vi "Get Reference for Specified Type (Project).vi"(8 "error in (no error)":errorcluster, 10 "Type to Find":string, 11 "Array of References":refnum<vi>[](array[refnum])) -> (0 "error out":errorcluster, 2 "Item Found":bool, 3 "Project Item":refnum<vi>)   [LabVIEW 2014, in "SPI Engine Scripting.lvlib"]
uses:
  SPI Engine Scripting.lvlib
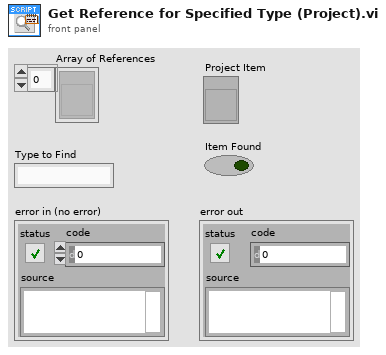
[diagram p1: front panel]
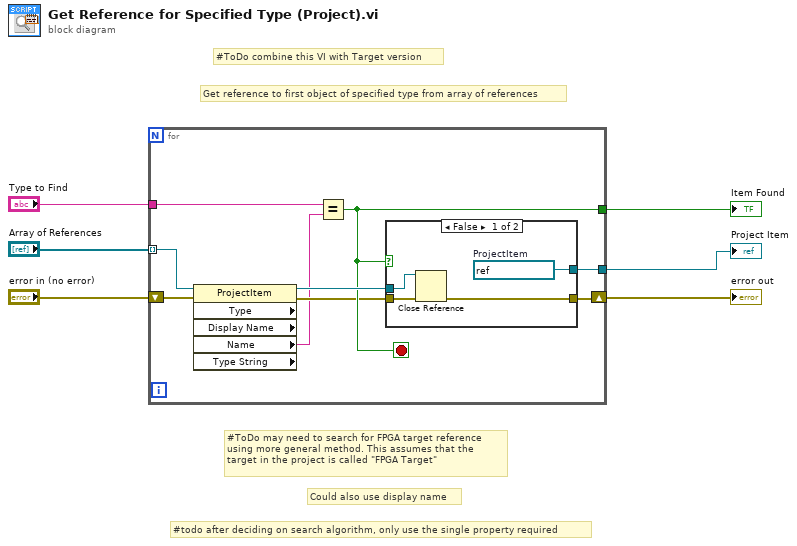
[diagram p0: block diagram]
diagram:
  # "#todo after deciding on search algorithm, only use the single property required"
  # "#ToDo combine this VI with Target version"
  # "#ToDo may need to search for FPGA target reference\nusing more general method. This assumes that the\ntarget in the project is called \"FPGA Target\""
  # "Could also use display name"
  # "Get reference to first object of specified type from array of references"
  n1 = for {
    tunnel: "Array of References" -> [w15] mode=indexing
    tunnel: "Type to Find" -> [w12]
    tunnel: [w11] -> w2
    shift-right: [w9] -> w3
    shift-left: "error in (no error)" -> [w14]
    tunnel: [w8] -> w1
    stop <- w11 stop-if-true
    n2 = property class="ProjectItem" props=["Type", "Display Name", "Name", "Type String"](reference=w15, error in=w14) -> (reference out=w13:refnum<vi>, error out=w10:errorcluster, "Name"=w7:string)  [unwired: 3 out]
    n3 = Equal?(x=w12, y=w7) -> (x = y?=w11:bool)
    n4 = case shown="False" w11 {
      tunnel: w13 -> [w17 w21]
      tunnel: [w16 w21] -> w8
      tunnel: w10 -> [w19 w20]
      tunnel: [w18 w20] -> w9
      frame False {
        w16 = refnum<vi> refnum  # ProjectItem
        n5 = Close Reference(reference=w17, error in (no error)=w19) -> (error out=w18:errorcluster)
      }
      frame True {
      }
    }
  }
  "error out" <- w3
  "Item Found" <- w2
  "Project Item" <- w1
